vi "Module Loop.vi"(8 "error in (no error)":errorcluster, 11 "Log Preparer Module in":refnum<class "Log Preparer Module.lvclass">) -> (0 "error out":errorcluster, 3 "Log Preparer Module out":refnum<class "Log Preparer Module.lvclass">)   [LabVIEW 2020, in "VolatusData.lvlib" / "Log Preparer Module.lvclass"]
uses:
  Log Preparer Module.lvclass
  C:/dev/lv20CE/relink/lv-volatus/Volatus/Module/Module.lvclass
  Volatus/Module/Module.lvclass
  Prep State.ctl
  Volatus/Module/Module.lvclass/Module.ctl
  Log Preparer Module.lvclass/Log Preparer Module.ctl
  <vilib>/Utility/error.llb/Error Cluster From Error Code.vi
  VolatusData.lvlib
  Volatus/Volatus.lvlib
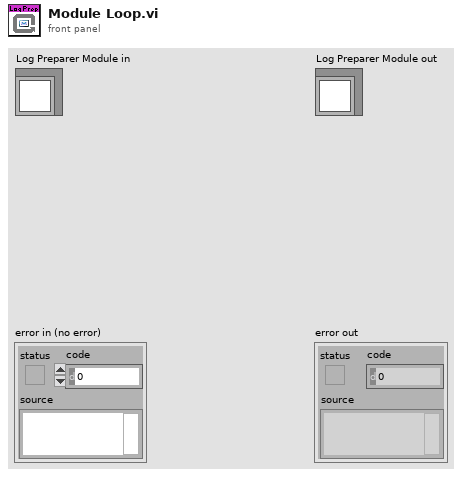
[diagram p1: front panel]
types:
  T1 = typedef "VolatusData.lvlib/Prep State.ctl" = enum16{"Unknown", "In Progress", "Success", "Failed"}
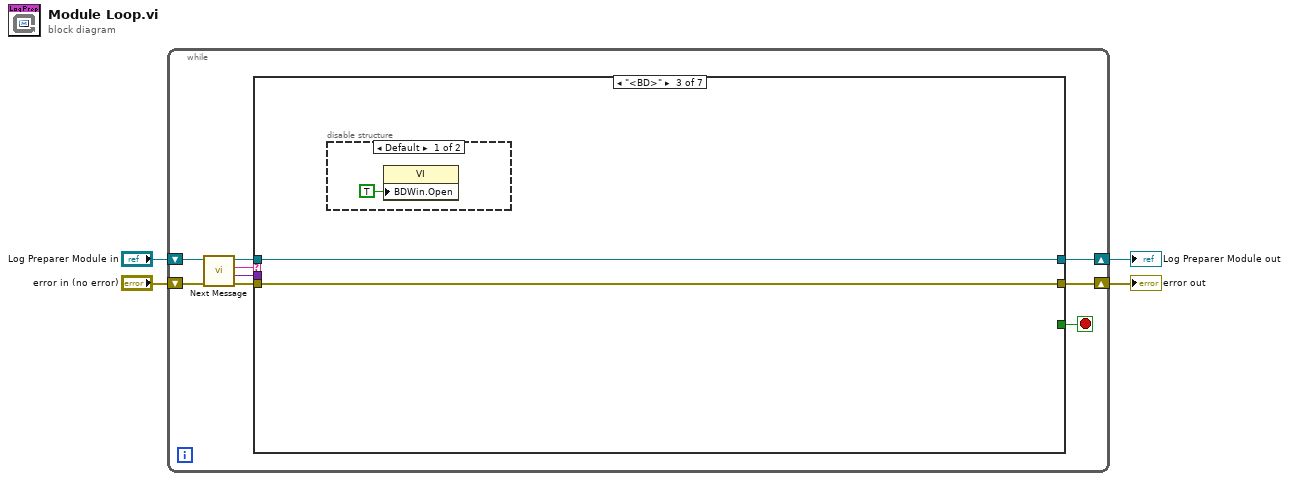
[diagram p0: block diagram]
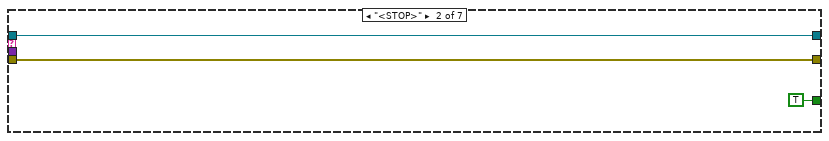
[diagram p3: hidden frame]
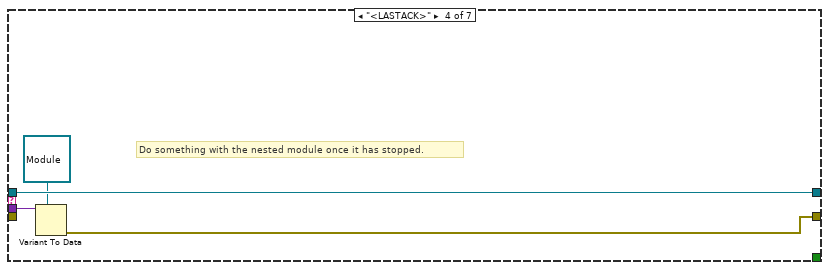
[diagram p5: hidden frame]
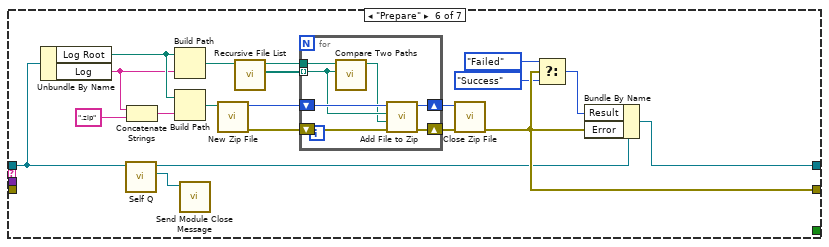
[diagram p7: hidden frame]
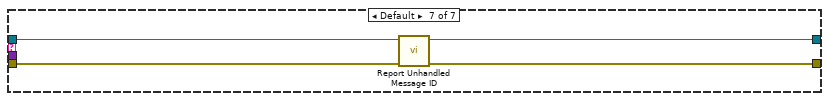
[diagram p8: hidden frame]
diagram:
  n1 = while {
    shift-right: [w8] -> w2
    shift-left: "Log Preparer Module in" -> [w13]
    shift-right: [w5] -> w1
    shift-left: "error in (no error)" -> [w12]
    stop <- w7 stop-if-true
    n2 = call "Next Message.vi"("error in (no error)"=w12, "Module in"=w13) -> ("error out"=w11:errorcluster, "Data"=w6:variant, "ID"=w10:string, "Module out"=w9:refnum<class "Log Preparer Module.lvclass">)  [unwired: 6 in]
    n3 = case shown="\"<BD>\"" w10 {
      tunnel: w11 -> [w14 w16 w19 _ w26 _ w58]
      tunnel: w9 -> [w15 w18 w20 w25 w27 w34 w56]
      tunnel: [w15 w18 w20 w25 w27 w30 w55] -> w8
      tunnel: [_ TRUE _ _ _ _ _] -> w7
      tunnel: w6 -> [_ _ _ w24 _ _ _]
      tunnel: [w14 w16 w19 w22 w26 w47 w57] -> w5
      frame "<CLOSE>" {
      }
      frame "<STOP>" {
      }
      frame "<BD>" {
        n4 = disable-structure shown="Default" {
          frame condition #0 (active) {
            n5 = property class="VI"("BDWin.Open"=TRUE ("Block Diagram Window:Open")) -> ()  [unwired: 2 in, 2 out]
          }
          frame condition #1 {
          }
        }
      }
      frame "<LASTACK>" {
        # "Do something with the nested module once it has stopped."
        n6 = Variant To Data(type=refnum<class "Module.lvclass"> refnum ("Volatus:Module"), Variant=w24) -> (error out=w22:errorcluster)  [unwired: 1 in, 1 out]
      }
      frame "<TIMEOUT>" {
        # "No message for this module was received in time"
      }
      frame "Prepare" {
        n7 = Unbundle By Name(w34) -> ("Log Root"=w44:path, "Log"=w38:string)
        n8 = call "Self Q.vi"("Module in"=w34) -> ("Self Q"=w28:refnum<class "MessageQ.lvclass">, "Module out"=w29:refnum<class "Log Preparer Module.lvclass">)  [unwired: 9 in]
        n9 = Concatenate Strings(w38, ".zip" ("string")) -> (w45:string)
        n10 = Build Path(base path=w44, name or relative path=w38) -> (appended path=w37:path)
        n11 = Build Path(base path=w44, name or relative path=w45) -> (appended path=w43:path)
        n12 = call "Send Module Close Message.vi"("MessageQ"=w28) -> ()  [unwired: 10 in, 1 out]
        n13 = call <vilib>:"New Zip File.vi"("target"=w43) -> ("error out"=w41:errorcluster, "zip file out"=w42:i64)  [unwired: 4 in, 1 out]
        n14 = call <vilib>:"Recursive File List.vi"("Folder Path"=w37) -> ("All Files in Dir"=w36:path[], "dup Folder Path"=w35:path)  [unwired: 6 in, 3 out]
        n15 = for {
          shift-right: [w52] -> w40
          shift-left: w42 -> [w54]
          shift-right: [w51] -> w39
          shift-left: w41 -> [w53]
          tunnel: w36 -> [w49] mode=indexing
          tunnel: w35 -> [w50]
          n16 = call <vilib>:"Compare Two Paths.vi"("Path 2"=w49, "Path 1"=w50) -> ("Relative Path from 1 to 2"=w48:path)  [unwired: 6 in, 3 out]
          n17 = call <vilib>:"Add File to Zip.vi"("error in (no error)"=w53, "destination path in zip"=w48, "source file path"=w49, "zip file in"=w54) -> ("error out"=w51:errorcluster, "zip file out"=w52:i64)  [unwired: 6 in]
        }
        n18 = call <vilib>:"Close Zip File.vi"("error in (no error)"=w39, "zip file in"=w40) -> ("error out"=w47:errorcluster)  [unwired: 5 in]
        n19 = Select(t=Prep_State."Failed" ("Result"), s=w47, f=Prep_State."Success" ("Result")) -> (s? t:f=w31:T1)
        n20 = Bundle By Name(cluster=w29, "Result"=w31, "Error"=w47) -> (w30:refnum<class "Log Preparer Module.lvclass">)
      }
      frame Default {
        n21 = call "Report Unhandled Message ID.vi"("error in (no error)"=w58, "Module in"=w56) -> ("error out"=w57:errorcluster, "Module out"=w55:refnum<class "Log Preparer Module.lvclass">)  [unwired: 8 in]
      }
    }
  }
  "error out" <- w1
  "Log Preparer Module out" <- w2
